vi "Write a and b.vi"(3 "b":dbl, 4 "a":dbl, 5 "Dual in":refnum<class "Dual.lvclass">) -> (2 "Dual out":refnum<class "Dual.lvclass">)   [LabVIEW 2020, in "Automatic Differentiation.lvlib" / "Dual.lvclass"]
uses:
  Dual.lvclass
  Dual.lvclass/Dual.ctl
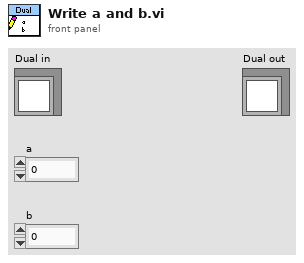
[diagram p1: front panel]
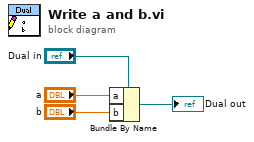
[diagram p0: block diagram]
diagram:
  n1 = Bundle By Name(cluster="Dual in", "a"="a", "b"="b") -> (→"Dual out":refnum<class "Dual.lvclass">)
